vi "Calculate Timeout.vi"(8 "error in (no error)":errorcluster, 10 "timeout ms":i32, 11 "t0":u32) -> (0 "error out":errorcluster, 4 "Elapsed?":bool, 5 "new timeout ms":i32)   [LabVIEW 2021, in "WebSockets.lvlib" / "WebSocket.lvclass"]
doc: "Calculates the remaining timeout since t0. Used to ensure calling VI doesn't exceed maximum timeout.\nWebSockets 2.0.1.40\nSam Sharp - MediaMongrels Ltd\nCopyright (c) 2019, MediaMongrels Ltd"
uses:
  WebSocket/WebSocket.lvclass
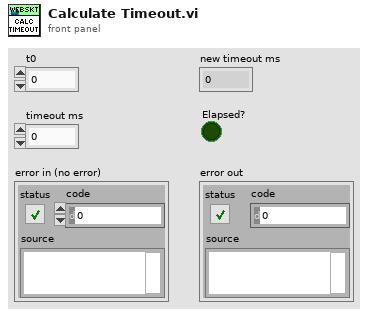
[diagram p1: front panel]
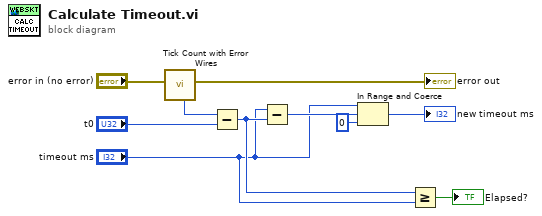
[diagram p0: block diagram]
diagram:
  n1 = call "Tick Count with Error Wires.vi"("error in (no error)"="error in (no error)") -> ("error out"=→"error out":errorcluster, "millisecond timer value"=w8:u32)  [unwired: 9 in]
  n2 = Subtract(x=w8, y="t0") -> (x-y=w3:i32)
  n3 = Subtract(x="timeout ms", y=w3) -> (x-y=w10:i32)
  n4 = In Range and Coerce(upper limit="timeout ms", x=w10, lower limit=0) -> (coerced(x)=→"new timeout ms":i32)  [unwired: 1 out]
  n5 = Greater Or Equal?(x=w3, y="timeout ms") -> (x >= y?=→"Elapsed?":bool)
